vi "EnqueueMessage(MsgName).vi"(5 "In Front? (F)":bool, 7 "Timeout (-1 ms)":i32, 8 "error in (no error)":errorcluster, 10 "Message Name":string, 11 "MessageQueue in":refnum<class "MessageQueue.lvclass">) -> (0 "error out":errorcluster, 3 "MessageQueue out":refnum<class "MessageQueue.lvclass">, 4 "Timed Out?":bool)   [LabVIEW 2017, in "LapDog.Messaging.v3.lvlib" / "MessageQueue.lvclass"]
doc: "Creates a dataless message object with the given name and adds it to the queue. By default the message is added to the rear of the queue. Set 'In Front?' to TRUE to add the message to the front of the queue.\n\nThis method executes regardless of the error in state."
uses:
  MessageQueue.lvclass
  Message/Message.lvclass
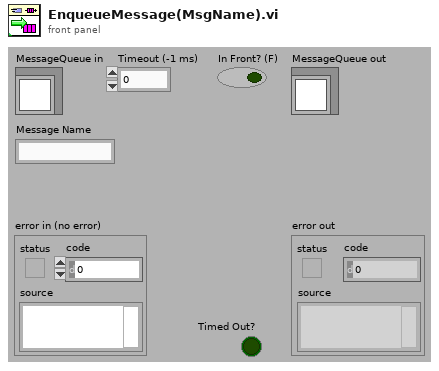
[diagram p1: front panel]
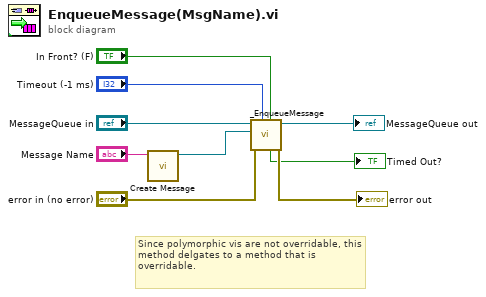
[diagram p0: block diagram]
diagram:
  # "Since polymorphic vis are not overridable, this method delgates to a method that is overridable."
  n1 = call "Create Message.vi"("Message Name"="Message Name") -> ("Message out"=w3:refnum<class "Message.lvclass">)  [unwired: 9 in, 1 out]
  n2 = call-dynamic "_EnqueueMessage.vi"("In Front? (F)"="In Front? (F)", "Timeout (-1 ms)"="Timeout (-1 ms)", "error in (no error)"="error in (no error)", "Message"=w3, "MessageQueue in"="MessageQueue in") -> ("error out"=→"error out":errorcluster, "MessageQueue out"=→"MessageQueue out":refnum<class "MessageQueue.lvclass">, "Timed Out?"=→"Timed Out?":bool)  [unwired: 4 in]
